vi "control_lasers_and_SMs_TIMING_TRUNCATED_LOOPS.vi"() -> ()   [LabVIEW 2021]
uses:
  <vilib>/DAQmx/write.llb/DAQmx Write (Analog 1D DBL NChan 1Samp).vi
  <vilib>/DAQmx/create/channels.llb/DAQmx Create Channel (AO-Voltage-Basic).vi
  <vilib>/DAQmx/miscellaneous.llb/DAQmx Fill In Error Info.vi
panel:
  in  "X2 (-10-10V) IV":dbl
  in  "Y2 (-10-10V) IV":dbl
  in  "X2 (-10-10V) III":dbl
  in  "Y2 (-10-10V) III":dbl
  in  "X2 (-10-10V) II":dbl
  in  "Y2 (-10-10V) II":dbl
  in  "Y2 (-10-10V)":dbl
  in  "X2 (-10-10V)":dbl
  in  "Continue Cycle?":bool
  out "Full Cycles":i32
  in  "Phase IV Duration (sec)":dbl=10.0 format="%.2f"
  in  "445 (0-10v) IV":dbl
  in  "488 (0-10v) IV":dbl
  in  "514 (0-10v) IV":dbl
  in  "561 (0-10v) IV":dbl
  in  "Blanking (0-10v) IV":dbl=10.0
  in  "X1 (-10-10V) IV":dbl
  in  "Y1 (-10-10V) IV":dbl
  out "Phase IV Iterations":i32
  in  "Phase III Duration (sec)":dbl=10.0 format="%.2f"
  in  "Phase II Duration (sec)":dbl=10.0 format="%.2f"
  in  "445 (0-10v) III":dbl
  in  "488 (0-10v) III":dbl
  in  "514 (0-10v) III":dbl
  in  "561 (0-10v) III":dbl
  in  "Blanking (0-10v) III":dbl=10.0
  in  "X1 (-10-10V) III":dbl
  in  "Y1 (-10-10V) III":dbl
  out "Phase III Iterations":i32
  in  "445 (0-10v) II":dbl
  in  "488 (0-10v) II":dbl
  in  "514 (0-10v) II":dbl
  in  "561 (0-10v) II":dbl
  in  "Blanking (0-10v) II":dbl=10.0
  in  "X1 (-10-10V) II":dbl
  in  "Y1 (-10-10V) II":dbl
  out "Phase II Iterations":i32
  out "Phase I Iterations":i32
  in  "Phase I Duration (sec)":dbl=10.0 format="%.2f"
  in  "Y1 (-10-10V)":dbl
  in  "X1 (-10-10V)":dbl
  in  "Blanking (0-10v)":dbl=10.0
  in  "561 (0-10v)":dbl
  in  "514 (0-10v)":dbl
  in  "488 (0-10v)":dbl
  in  "445 (0-10v)":dbl
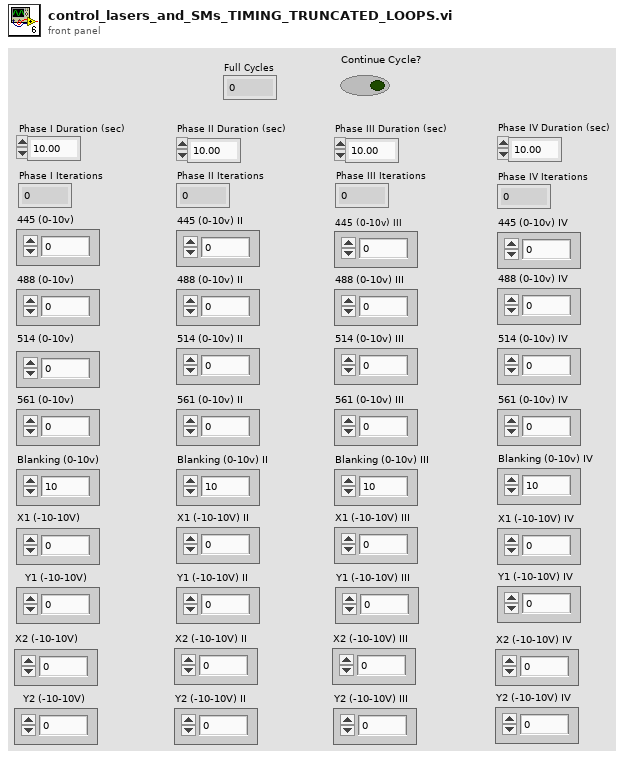
[diagram p1: front panel]
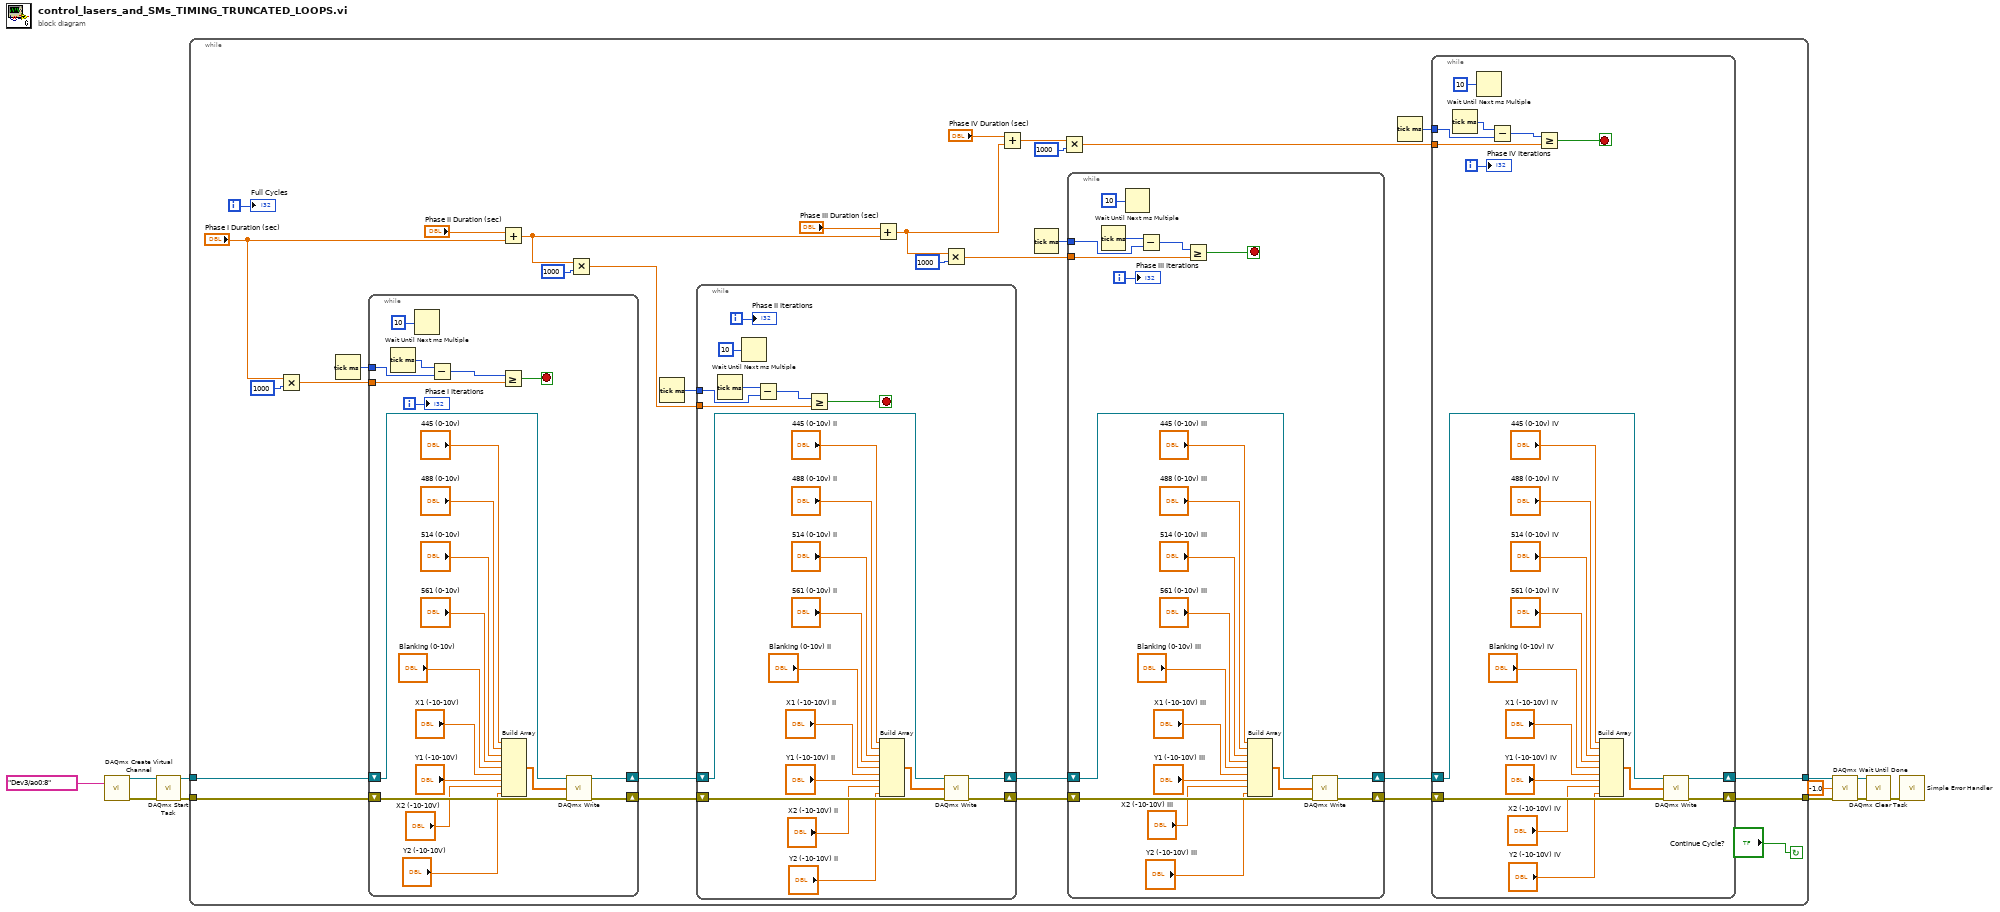
[diagram p0: block diagram]
diagram:
  n1 = call-poly <vilib>:"DAQmx Create Virtual Channel.vi"("physical channels"=tag "Dev3/ao0:8") -> ("task out"=w4:refnum<k21>, "error out"=w3:errorcluster)  [unwired: 13 in]
  n2 = call <vilib>:"DAQmx Start Task.vi"("task/channels in"=w4, "error in"=w3) -> ("task out"=w2:refnum<k21>, "error out"=w1:errorcluster)  [unwired: 12 in]
  n3 = while {
    tunnel: [w19] -> w7
    tunnel: [w18] -> w6
    tunnel: w2 -> [w14]
    tunnel: w1 -> [w13]
    i -> [w15]
    stop <- "Continue Cycle?" continue-if-true
    n4 = Multiply(x="Phase I Duration (sec)", y=1000) -> (x*y=w40:dbl)
    n5 = Tick Count (ms)() -> (millisecond timer value=w41:u32)
    n6 = while {
      shift-right: [w103] -> w33
      shift-left: w14 -> [w105]
      shift-right: [w102] -> w32
      shift-left: w13 -> [w104]
      tunnel: w41 -> [w92]
      tunnel: w40 -> [w88]
      i -> [w93]
      stop <- w89 stop-if-true
      n7 = Tick Count (ms)() -> (millisecond timer value=w91:u32)
      n8 = Wait Until Next ms Multiple(millisecond multiple=10) -> ()  [unwired: 1 out]
      n9 = Subtract(x=w91, y=w92) -> (x-y=w90:u32)
      n10 = Greater Or Equal?(x=w90, y=w88) -> (x >= y?=w89:bool)
      n11 = Build Array("445 (0-10v)", "488 (0-10v)", "514 (0-10v)", "561 (0-10v)", "Blanking (0-10v)", "X1 (-10-10V)", "Y1 (-10-10V)", "X2 (-10-10V)", "Y2 (-10-10V)") -> (w101:dbl[])
      n12 = call-poly <vilib>:"DAQmx Write.vi"("task/channels in"=w105, "data"=w101, "error in"=w104) -> ("task out"=w103:refnum<k21>, "error out"=w102:errorcluster)  [unwired: 10 in, 1 out]
      "Phase I Iterations" <- w93
    }
    n13 = Add(x="Phase II Duration (sec)", y="Phase I Duration (sec)") -> (x+y=w27:dbl)
    n14 = Multiply(x=w27, y=1000) -> (x*y=w37:dbl)
    n15 = Tick Count (ms)() -> (millisecond timer value=w38:u32)
    n16 = while {
      shift-right: [w82] -> w30
      shift-left: w33 -> [w84]
      shift-right: [w81] -> w31
      shift-left: w32 -> [w83]
      tunnel: w38 -> [w71]
      tunnel: w37 -> [w67]
      i -> [w72]
      stop <- w68 stop-if-true
      n17 = Tick Count (ms)() -> (millisecond timer value=w70:u32)
      n18 = Wait Until Next ms Multiple(millisecond multiple=10) -> ()  [unwired: 1 out]
      n19 = Subtract(x=w70, y=w71) -> (x-y=w69:u32)
      n20 = Greater Or Equal?(x=w69, y=w67) -> (x >= y?=w68:bool)
      n21 = Build Array("445 (0-10v) II", "488 (0-10v) II", "514 (0-10v) II", "561 (0-10v) II", "Blanking (0-10v) II", "X1 (-10-10V) II", "Y1 (-10-10V) II", "X2 (-10-10V) II", "Y2 (-10-10V) II") -> (w80:dbl[])
      n22 = call-poly <vilib>:"DAQmx Write.vi"("task/channels in"=w84, "data"=w80, "error in"=w83) -> ("task out"=w82:refnum<k21>, "error out"=w81:errorcluster)  [unwired: 10 in, 1 out]
      "Phase II Iterations" <- w72
    }
    n23 = Add(x="Phase III Duration (sec)", y=w27) -> (x+y=w24:dbl)
    n24 = Multiply(x=w24, y=1000) -> (x*y=w34:dbl)
    n25 = Add(x="Phase IV Duration (sec)", y=w24) -> (x+y=w23:dbl)
    n26 = Tick Count (ms)() -> (millisecond timer value=w35:u32)
    n27 = Multiply(x=w23, y=1000) -> (x*y=w25:dbl)
    n28 = while {
      shift-right: [w61] -> w21
      shift-left: w30 -> [w63]
      shift-right: [w60] -> w20
      shift-left: w31 -> [w62]
      tunnel: w35 -> [w50]
      tunnel: w34 -> [w46]
      i -> [w51]
      stop <- w47 stop-if-true
      n29 = Tick Count (ms)() -> (millisecond timer value=w49:u32)
      n30 = Wait Until Next ms Multiple(millisecond multiple=10) -> ()  [unwired: 1 out]
      n31 = Subtract(x=w49, y=w50) -> (x-y=w48:u32)
      n32 = Greater Or Equal?(x=w48, y=w46) -> (x >= y?=w47:bool)
      n33 = Build Array("445 (0-10v) III", "488 (0-10v) III", "514 (0-10v) III", "561 (0-10v) III", "Blanking (0-10v) III", "X1 (-10-10V) III", "Y1 (-10-10V) III", "X2 (-10-10V) III", "Y2 (-10-10V) III") -> (w59:dbl[])
      n34 = call-poly <vilib>:"DAQmx Write.vi"("task/channels in"=w63, "data"=w59, "error in"=w62) -> ("task out"=w61:refnum<k21>, "error out"=w60:errorcluster)  [unwired: 10 in, 1 out]
      "Phase III Iterations" <- w51
    }
    n35 = Tick Count (ms)() -> (millisecond timer value=w16:u32)
    n36 = while {
      shift-right: [w124] -> w19
      shift-left: w21 -> [w126]
      shift-right: [w123] -> w18
      shift-left: w20 -> [w125]
      tunnel: w16 -> [w113]
      tunnel: w25 -> [w109]
      i -> [w114]
      stop <- w110 stop-if-true
      n37 = Tick Count (ms)() -> (millisecond timer value=w112:u32)
      n38 = Wait Until Next ms Multiple(millisecond multiple=10) -> ()  [unwired: 1 out]
      n39 = Subtract(x=w112, y=w113) -> (x-y=w111:u32)
      n40 = Greater Or Equal?(x=w111, y=w109) -> (x >= y?=w110:bool)
      n41 = Build Array("445 (0-10v) IV", "488 (0-10v) IV", "514 (0-10v) IV", "561 (0-10v) IV", "Blanking (0-10v) IV", "X1 (-10-10V) IV", "Y1 (-10-10V) IV", "X2 (-10-10V) IV", "Y2 (-10-10V) IV") -> (w122:dbl[])
      n42 = call-poly <vilib>:"DAQmx Write.vi"("task/channels in"=w126, "data"=w122, "error in"=w125) -> ("task out"=w124:refnum<k21>, "error out"=w123:errorcluster)  [unwired: 10 in, 1 out]
      "Phase IV Iterations" <- w114
    }
    "Full Cycles" <- w15
  }
  n43 = call <vilib>:"DAQmx Wait Until Done.vi"("task/channels in"=w7, "timeout (sec)"=-1.0, "error in"=w6) -> ("task out"=w10:refnum<k21>, "error out"=w9:errorcluster)  [unwired: 11 in]
  n44 = call <vilib>:"DAQmx Clear Task.vi"("task in"=w10, "error in"=w9) -> ("error out"=w11:errorcluster)  [unwired: 13 in]
  n45 = call <vilib>:"Simple Error Handler.vi"("error in (no error)"=w11) -> ()  [unwired: 4 in, 5 out]
